vi "Get Server Internal UEs.vi"(11 "OOP Server in":refnum<class "TestDataMarshal.lvclass">) -> (2 "Server Internal UEs":T1, 3 "OOP Server out":refnum<class "TestDataMarshal.lvclass">)   [LabVIEW 2019, in "TestDataMarshal.lvlib" / "TestDataMarshal.lvclass"]
uses:
  TestDataMarshal.lvclass
  typeDefs/Server Internal UEs.ctl
  typeDefs/Server Internal Message.ctl
  TestDataMarshal.lvclass/TestDataMarshal.ctl
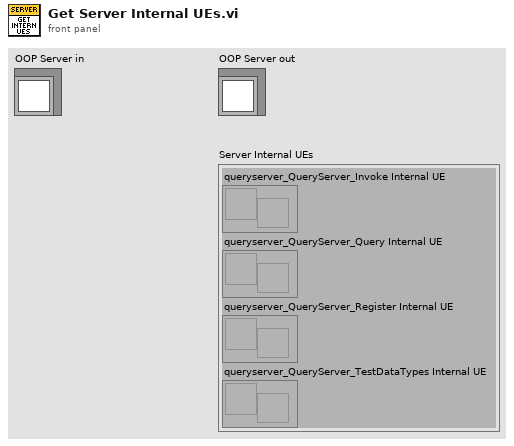
[diagram p1: front panel]
types:
  T1 = typedef "TestDataMarshal.lvlib/TestDataMarshal.lvclass/Server Internal UEs.ctl" = cluster{"queryserver_QueryServer_Invoke Internal UE":refnum<user-event>, "queryserver_QueryServer_Query Internal UE":refnum<user-event>, "queryserver_QueryServer_Register Internal UE":refnum<user-event>, "queryserver_QueryServer_TestDataTypes Internal UE":refnum<user-event>}
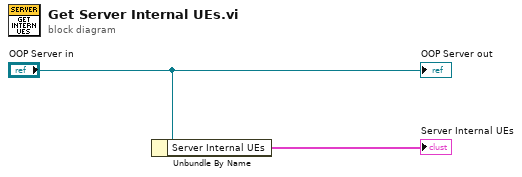
[diagram p0: block diagram]
diagram:
  n1 = Unbundle By Name("OOP Server in") -> ("Server Internal UEs"=→"Server Internal UEs":T1)
  "OOP Server out" <- "OOP Server in"
